vi "GetDriverConfig.vi"(0 "TestConfigFileName":string="Eggy55W.hwc") -> (4 "OUT VISA":string[][](array[string]), 6 "初始化结果信息":string[](array[string]), 8 "初始化结果":bool[](array[boolean]), 10 "OUT VISA NAME":string[](array[string]))   [LabVIEW 2018]
uses:
  Subvi/Global.vi
  <vilib>/Instr/_visa.llb/VISA Configure Serial Port (Instr).vi
panel:
  out "元素":string
  out "数字":dbl
  out "字符串 5":string
  out "字符串 4":string
  out "字符串 3":string
  out "字符串 2":string
  out "数组":string[](array[string])
  out "GPIB_1":refnum<visa-resource-name>
  out "*(类型 *) &x":refnum<visa-resource-name>
  out "字符串":string
  out "滑动杆":u8(slide) scale=0.0..100.0
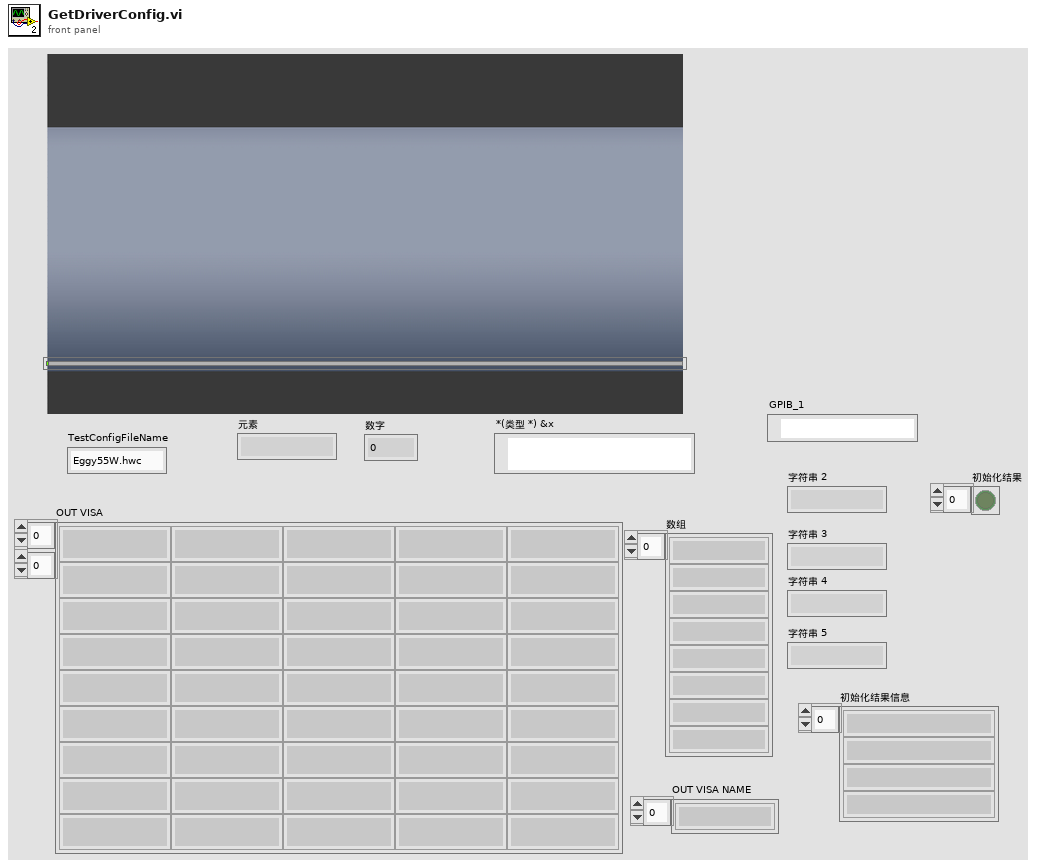
[diagram p1: front panel]
types:
  T1 = enum16{"open", "replace", "create", "open or create", "replace or create", "replace or create with confirmation"}
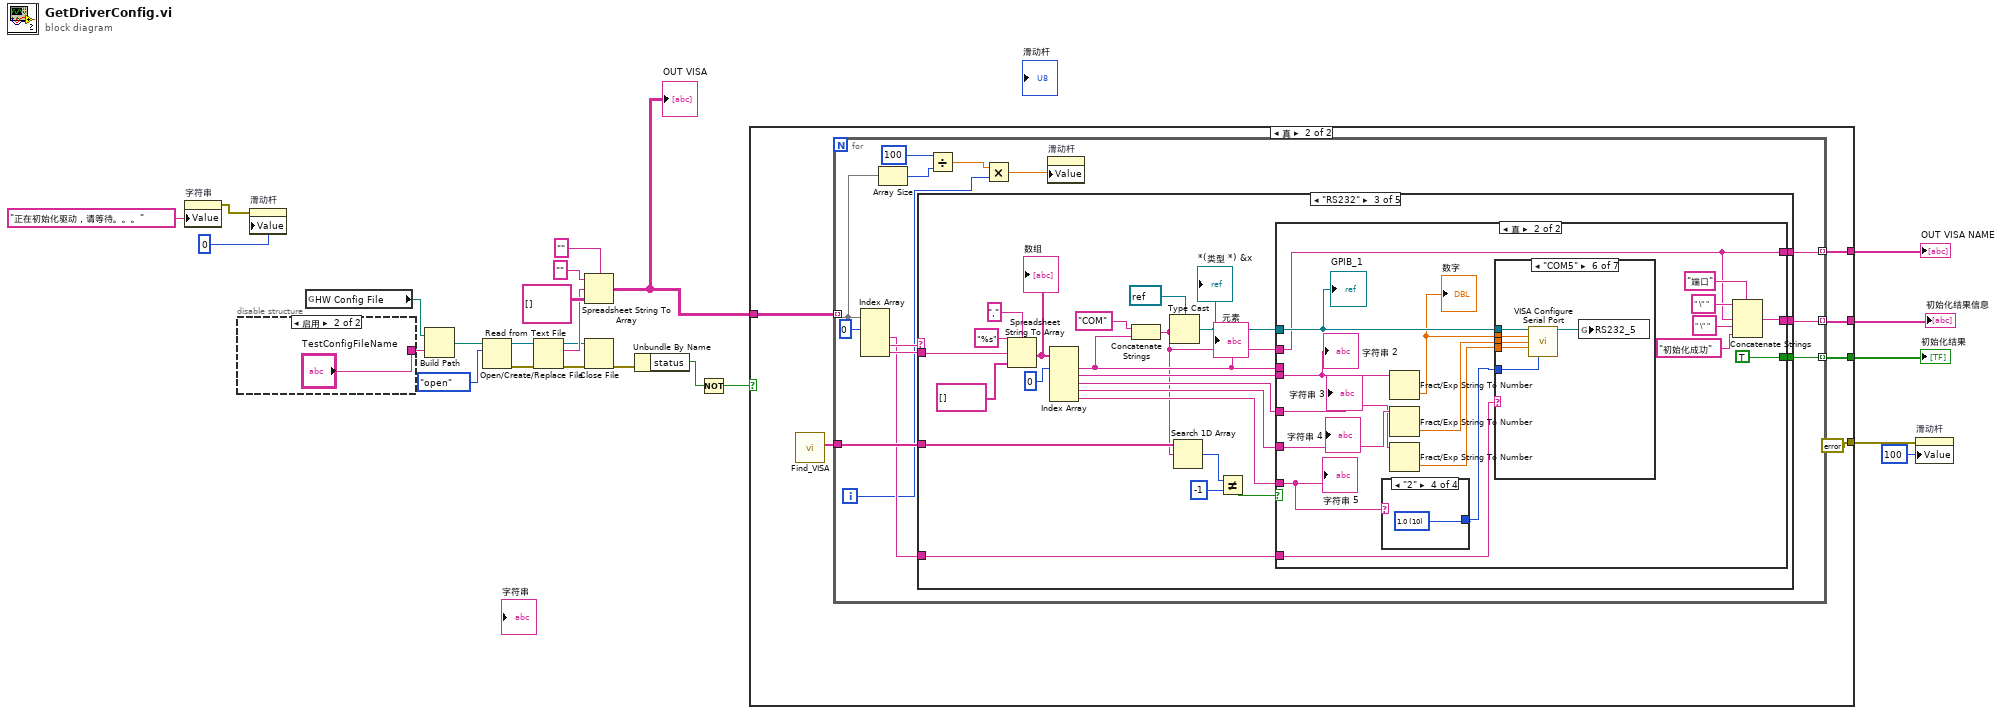
[diagram p0: block diagram]
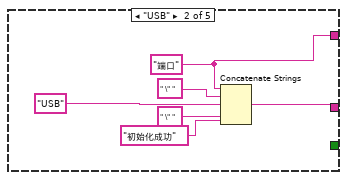
[diagram p4: hidden frame]
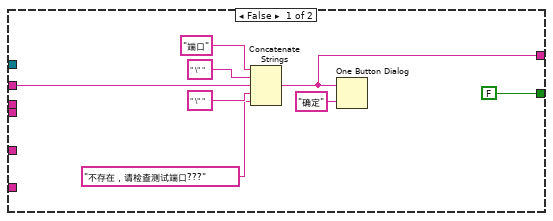
[diagram p5: hidden frame]
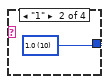
[diagram p7: hidden frame]
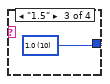
[diagram p8: hidden frame]
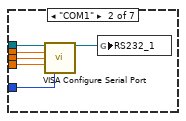
[diagram p10: hidden frame]
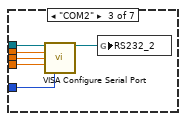
[diagram p11: hidden frame]
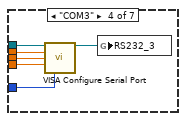
[diagram p12: hidden frame]
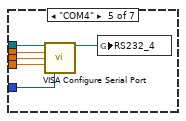
[diagram p13: hidden frame]
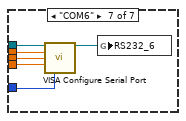
[diagram p14: hidden frame]
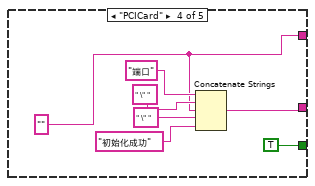
[diagram p15: hidden frame]
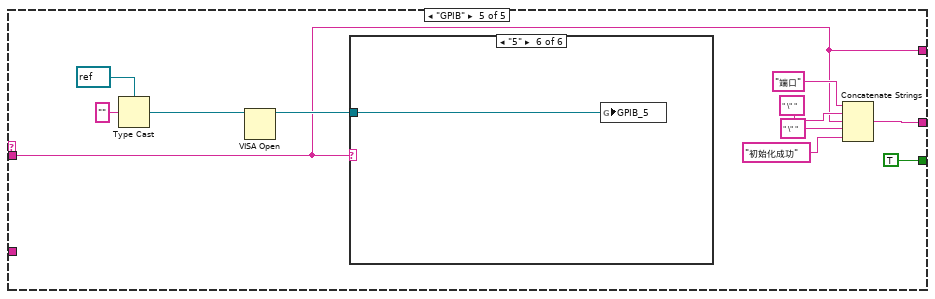
[diagram p16: hidden frame]
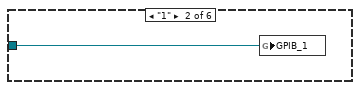
[diagram p18: hidden frame]
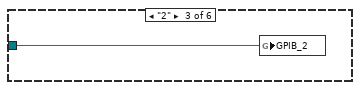
[diagram p19: hidden frame]
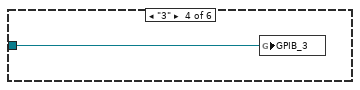
[diagram p20: hidden frame]
diagram:
  n1 = property on="字符串" class="Str"("Value"="正在初始化驱动，请等待。。。" ("字符串")) -> (error out=w2:errorcluster)  [unwired: 2 in, 1 out]
  n2 = disable-structure shown="启用" {
    disable-tunnel: ["DEMO3.hwc" ("element") "TestConfigFileName"] -> w13
    frame Disabled {
    }
    frame Enabled {
    }
  }
  n3 = property on="滑动杆" class="Slide (严格)"(error in=w2, "Value"=u8 0 ("滑动杆")) -> ()  [unwired: 1 in, 2 out]
  n4 = global read "Global.vi" "HW Config File"() -> (w14:path)
  n5 = Build Path(base path=w14, name or relative path=w13) -> (appended path=w15:path)
  n6 = Open/Create/Replace File(file path (use dialog)=w15, operation (0:open)=T1."open") -> (refnum out=w16:refnum<file>, error out=w18:errorcluster)  [unwired: 1 in, 4 out]
  n7 = Read from Text File(file (use dialog)=w16, error in=w18) -> (refnum out=w17:refnum<file>, text=w21:string, error out=w19:errorcluster)  [unwired: 3 out]
  n8 = Spreadsheet String To Array(delimiter (Tab)="", format string="", spreadsheet string=w21, array type (2D Dbl)=string[][] []) -> (array=w12:string[][])
  "OUT VISA" <- w12
  n9 = Close File(refnum=w17, error in=w19) -> (error out=w4:errorcluster)  [unwired: 1 out]
  n10 = Unbundle By Name(w4) -> ("status"=w8:bool)
  n11 = Not(x=w8) -> (.not. x?=w7:bool)
  n12 = case shown="真" w7 {
    tunnel: w12 -> [_ w32]
    tunnel: [_ w30] -> w11
    tunnel: [_ w29] -> w10
    tunnel: [_ w28] -> w9
    tunnel: [_ errorcluster {"status"=FALSE, "code"=0, "source"=""} ("错误输出")] -> w6
    frame False {
    }
    frame True {
      n13 = call "Find_VISA.vi"() -> ("Com port list"=w31:string[])  [unwired: 11 in]
      n14 = for {
        tunnel: w32 -> [w38] mode=indexing
        tunnel: w31 -> [w43]
        tunnel: [w42] -> w29 mode=indexing
        tunnel: [w41] -> w30 mode=indexing
        tunnel: [w40] -> w28 mode=indexing
        i -> [w34]
        n15 = Index Array(array=w38, index #1=0 ("索引")) -> (element #2=w39:string, element #3=w45:string, element #4=w44:string)  [unwired: 3 in, 1 out]
        n16 = Array Size(array=w38) -> (size(s)=w36:i32)
        n17 = case shown="\"RS232\"" w45 {
          tunnel: w44 -> [_ _ w72 _ w147]
          tunnel: w43 -> [_ _ w62 _ _]
          tunnel: [_ _ w57 TRUE ("true") TRUE ("true")] -> w42
          tunnel: [_ w49 w56 w142 w150] -> w41
          tunnel: [_ w47 w55 w140 w147] -> w40
          tunnel: w39 -> [_ _ w53 _ _]
          frame "假", Default {
          }
          frame "USB" {
            w47 = "端口" ("消息")
            n18 = Concatenate Strings(w47, " \" " ("字符串"), "USB" ("字符串"), " \" " ("字符串"), "初始化成功" ("字符串")) -> (w49:string)
          }
          frame "RS232" {
            n19 = Spreadsheet String To Array(delimiter (Tab)="," ("分隔符(Tab)"), format string="%s" ("格式字符串"), spreadsheet string=w72, array type (2D Dbl)=string[] []) -> (array=w71:string[])
            "数组" <- w71
            n20 = Index Array(array=w71, index #1=0 ("索引")) -> (element #1=w61:string, element #2=w66:string, element #3=w65:string, element #4=w64:string, element #5=w63:string)  [unwired: 4 in]
            "元素" <- w61
            n21 = Concatenate Strings("COM" ("字符串"), w61) -> (w54:string)
            n22 = Type Cast(type=refnum<visa-resource-name> refnum ("GPIB_1"), x=w54) -> (*(type *) &x=w67:refnum<visa-resource-name>)
            "*(类型 *) &x" <- w67
            n23 = Search 1D Array(1D array=w62, element=w54) -> (index of element=w60:i32)  [unwired: 1 in]
            n24 = Not Equal?(x=w60, y=-1) -> (x != y?=w58:bool)
            n25 = case shown="真" w58 {
              tunnel: w61 -> [_ _]
              tunnel: w67 -> [_ w100]
              tunnel: w66 -> [_ w88]
              tunnel: w65 -> [_ w86]
              tunnel: w64 -> [_ w87]
              tunnel: w63 -> [_ w85]
              tunnel: w54 -> [w82 w90]
              tunnel: [FALSE ("true") TRUE ("true")] -> w57
              tunnel: [w76 w92] -> w56
              tunnel: [_ w90] -> w55
              tunnel: w53 -> [_ w84]
              frame False {
                n26 = Concatenate Strings("端口" ("消息"), " \" " ("字符串"), w82, " \" " ("字符串"), "不存在，请检查测试端口???") -> (w76:string)
                n27 = One Button Dialog(message=w76, button name ("OK")="确定" ("按钮名称（“确定”）")) -> ()  [unwired: 1 out]
              }
              frame True {
                n28 = case shown="\"2\"" w85 {
                  tunnel: [_ w101 w102 w103] -> w89
                  frame "假", Default {
                  }
                  frame "1" {
                    w101 = u16 10 items=["1.0"=10, "1.5"=15, "2.0"=20] ("stop bits (10: 1 bit)")
                  }
                  frame "1.5" {
                    w102 = u16 10 items=["1.0"=10, "1.5"=15, "2.0"=20] ("stop bits (10: 1 bit)")
                  }
                  frame "2" {
                    w103 = u16 10 items=["1.0"=10, "1.5"=15, "2.0"=20] ("stop bits (10: 1 bit)")
                  }
                }
                n29 = Fract/Exp String To Number(string=w88) -> (number=w99:dbl)  [unwired: 3 in, 1 out]
                "数字" <- w99
                n30 = Fract/Exp String To Number(string=w87) -> (number=w98:dbl)  [unwired: 3 in, 1 out]
                n31 = Fract/Exp String To Number(string=w86) -> (number=w97:dbl)  [unwired: 3 in, 1 out]
                n32 = case shown="\"COM5\"" w84 {
                  tunnel: w100 -> [_ w109 w115 w121 w127 w133 w139]
                  tunnel: w99 -> [_ w108 w114 w120 w126 w132 w138]
                  tunnel: w98 -> [_ w107 w113 w119 w125 w131 w137]
                  tunnel: w97 -> [_ w106 w112 w118 w124 w130 w136]
                  tunnel: w89 -> [_ w105 w111 w117 w123 w129 w135]
                  frame "假", Default {
                  }
                  frame "COM1" {
                    n33 = call-poly "VISA Configure Serial Port"("VISA resource name"=w109, "baud rate (9600)"=w108, "data bits (8)"=w107, "parity (0:none)"=w106, "stop bits (10: 1 bit)"=w105) -> ("VISA resource name out"=w104:refnum<visa-resource-name>)  [unwired: 9 in, 1 out]
                    n34 = global write "Global.vi" "RS232_1"(w104) -> ()
                  }
                  frame "COM2" {
                    n35 = call-poly "VISA Configure Serial Port"("VISA resource name"=w115, "baud rate (9600)"=w114, "data bits (8)"=w113, "parity (0:none)"=w112, "stop bits (10: 1 bit)"=w111) -> ("VISA resource name out"=w110:refnum<visa-resource-name>)  [unwired: 9 in, 1 out]
                    n36 = global write "Global.vi" "RS232_2"(w110) -> ()
                  }
                  frame "COM3" {
                    n37 = call-poly "VISA Configure Serial Port"("VISA resource name"=w121, "baud rate (9600)"=w120, "data bits (8)"=w119, "parity (0:none)"=w118, "stop bits (10: 1 bit)"=w117) -> ("VISA resource name out"=w116:refnum<visa-resource-name>)  [unwired: 9 in, 1 out]
                    n38 = global write "Global.vi" "RS232_3"(w116) -> ()
                  }
                  frame "COM4" {
                    n39 = call-poly "VISA Configure Serial Port"("VISA resource name"=w127, "baud rate (9600)"=w126, "data bits (8)"=w125, "parity (0:none)"=w124, "stop bits (10: 1 bit)"=w123) -> ("VISA resource name out"=w122:refnum<visa-resource-name>)  [unwired: 9 in, 1 out]
                    n40 = global write "Global.vi" "RS232_4"(w122) -> ()
                  }
                  frame "COM5" {
                    n41 = call-poly "VISA Configure Serial Port"("VISA resource name"=w133, "baud rate (9600)"=w132, "data bits (8)"=w131, "parity (0:none)"=w130, "stop bits (10: 1 bit)"=w129) -> ("VISA resource name out"=w128:refnum<visa-resource-name>)  [unwired: 9 in, 1 out]
                    n42 = global write "Global.vi" "RS232_5"(w128) -> ()
                  }
                  frame "COM6" {
                    n43 = call-poly "VISA Configure Serial Port"("VISA resource name"=w139, "baud rate (9600)"=w138, "data bits (8)"=w137, "parity (0:none)"=w136, "stop bits (10: 1 bit)"=w135) -> ("VISA resource name out"=w134:refnum<visa-resource-name>)  [unwired: 9 in, 1 out]
                    n44 = global write "Global.vi" "RS232_6"(w134) -> ()
                  }
                }
                n45 = Concatenate Strings("端口" ("消息"), " \" " ("字符串"), w90, " \" " ("字符串"), "初始化成功" ("字符串")) -> (w92:string)
                "GPIB_1" <- w100
                "字符串 2" <- w88
                "字符串 3" <- w86
                "字符串 4" <- w87
                "字符串 5" <- w85
              }
            }
          }
          frame "PCICard" {
            w140 = "" ("字符串")
            n46 = Concatenate Strings("端口" ("消息"), " \" " ("字符串"), w140, " \" " ("字符串"), "初始化成功" ("字符串")) -> (w142:string)
          }
          frame "GPIB" {
            n47 = Type Cast(type=refnum<visa-resource-name> refnum ("GPIB_1"), x="") -> (*(type *) &x=w155:refnum<visa-resource-name>)
            n48 = VISA Open(VISA resource name=w155) -> (VISA resource name=w154:refnum<visa-resource-name>)  [unwired: 4 in, 1 out]
            n49 = case shown="\"5\"" w147 {
              tunnel: w154 -> [_ w158 w159 w160 w161 w162]
              frame "假", Default {
              }
              frame "1" {
                n50 = global write "Global.vi" "GPIB_1"(w158) -> ()
              }
              frame "2" {
                n51 = global write "Global.vi" "GPIB_2"(w159) -> ()
              }
              frame "3" {
                n52 = global write "Global.vi" "GPIB_3"(w160) -> ()
              }
              frame "4" {
                n53 = global write "Global.vi" "GPIB_4"(w161) -> ()
              }
              frame "5" {
                n54 = global write "Global.vi" "GPIB_5"(w162) -> ()
              }
            }
            n55 = Concatenate Strings("端口" ("消息"), " \" " ("字符串"), w147, " \" " ("字符串"), "初始化成功" ("字符串")) -> (w150:string)
          }
        }
        n56 = Divide(x=100, y=w36) -> (x/y=w35:dbl)
        n57 = Multiply(x=w35, y=w34) -> (x*y=w33:dbl)
        n58 = property on="滑动杆" class="Slide (严格)"("Value"=w33) -> ()  [unwired: 2 in, 2 out]
      }
    }
  }
  "初始化结果信息" <- w11
  "初始化结果" <- w10
  "OUT VISA NAME" <- w9
  n59 = property on="滑动杆" class="Slide (严格)"(error in=w6, "Value"=u8 100 ("滑动杆")) -> ()  [unwired: 1 in, 2 out]
